vi "SearchEachElFrom1DToEveryIdxIn2D Modified.vi"(8 "This Array":u64[](array[numeric]), 11 "2D Target Array":i32[][](array[numeric])) -> (0 "Map matching":map{string, i32}(c390), 3 "Matching array":u64[](array[numeric]))   [LabVIEW 2023]
panel:
  out "2D Size":i32
  out "1D Size":i32
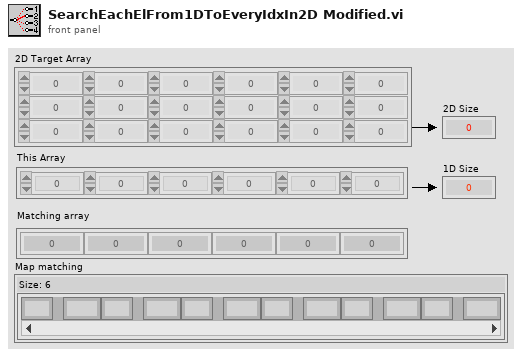
[diagram p1: front panel]
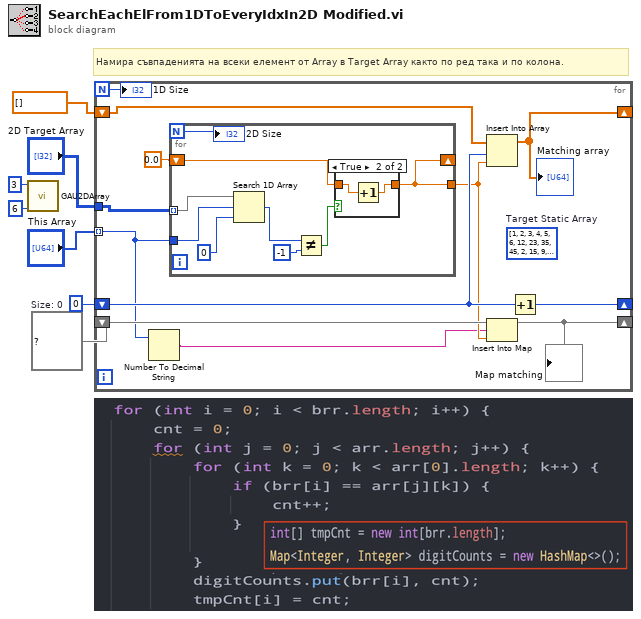
[diagram p0: block diagram]
diagram:
  w1 = map{string, i32} {}  # Size: 0
  # "Намира съвпаденията на всеки елемент от Array в Target Array както по ред така и по колона."
  n1 = call "GAU2DArray.vi"("Colums"=6, "Rows"=3) -> ()  [unwired: 8 in, 2 out]
  n2 = for {
    N -> [w8]
    tunnel: "This Array" -> [w10] mode=indexing
    tunnel: "2D Target Array" -> [w19]
    shift-right: [w17] -> _
    shift-left: dbl[] [] -> [w16]
    shift-right: [w15] -> _
    shift-left: u64 0 -> [w14]
    shift-right: [w13] -> _
    shift-left: w1 -> [w12]
    (unwired) u64[][] [[1, 2, 3, 4, 5, 6], [12, 23, 35, 45, 2, 15], [9, 3, 14, 5, 6, 7]]  # Target Static Array
    n3 = Number To Decimal String(number=w10) -> (decimal integer string=w9:string)  [unwired: 1 in]
    n4 = for {
      N -> [w20]
      tunnel: w19 -> [w28] mode=indexing
      tunnel: w10 -> [w27]
      shift-right: [w21] -> _
      shift-left: 0.0 -> [w23]
      tunnel: [w21] -> w11
      n5 = Search 1D Array(1D array=w28, element=w27, start index (0)=0) -> (index of element=w26:i32)
      n6 = Not Equal?(x=w26, y=-1) -> (x != y?=w24:bool)
      n7 = case shown="True" w24 {
        tunnel: [w29 w31] -> w21
        tunnel: w23 -> [w29 w30]
        frame False {
        }
        frame True {
          n8 = Increment(x=w30) -> (x+1=w31:dbl)
        }
      }
      "2D Size" <- w20
    }
    n9 = Insert Into Array "Insert Into Array"(array=w16, index=w14, new element=w11) -> (w17:dbl[])
    "Matching array" <- w17
    n10 = Insert Into Map(map in=w12, key=w9, value=w11) -> (map out=w13:map{string, i32})  [unwired: 2 out]
    "Map matching" <- w13
    n11 = Increment(x=w14) -> (x+1=w15:u64)
    "1D Size" <- w8
  }
